vi "Mavlink Initialize.vi"(7 "error in":errorcluster, 9 "Packet Sequence In":u8, 10 "VISA in":refnum<visa-resource-name>) -> (0 "Error Out":errorcluster, 2 "Packet Sequence Out":u8, 3 "VISA resource name Out":refnum<visa-resource-name>)   [LabVIEW 2023]
panel:
  out "Send Data":string
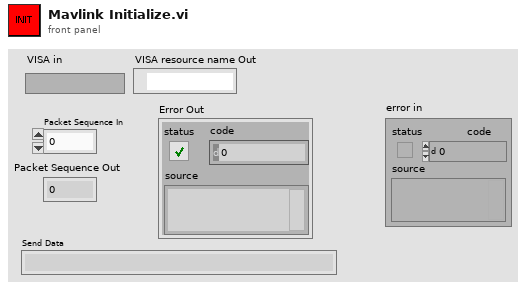
[diagram p1: front panel]
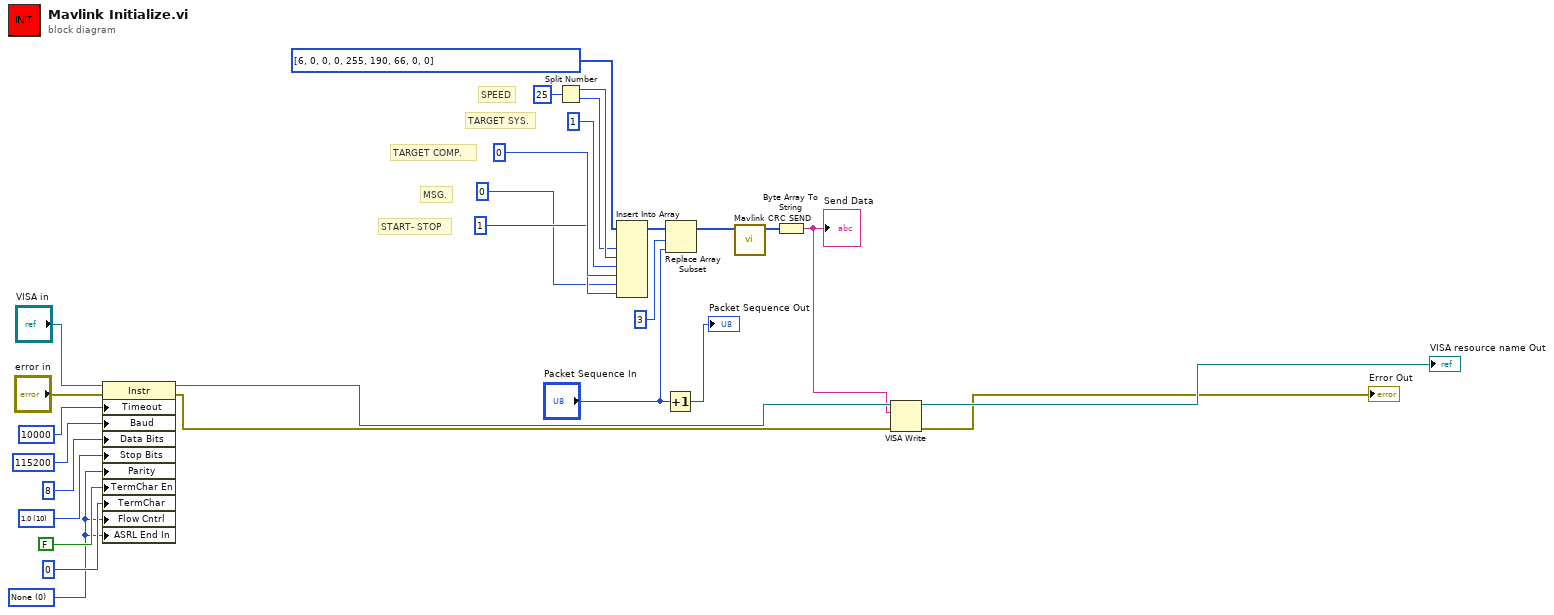
[diagram p0: block diagram]
diagram:
  w20 = u16 0 items=["None", "Last Bit", "TermChar"] ("Serial Settings:End Mode for Reads")
  w23 = u16 10 items=["1.0"=10, "1.5"=15, "2.0"=20] ("Serial Settings:Stop Bits")
  # "START- STOP"
  # "TARGET COMP."
  # "TARGET SYS."
  # "SPEED"
  # "MSG."
  n1 = property class="Instr"(reference="VISA in", error in="error in", "Timeout"=u32 10000 ("General Settings:Timeout Value"), "Baud"=u32 115200 ("Serial Settings:Baud Rate"), "Data Bits"=u16 8 ("Serial Settings:Data Bits"), "Stop Bits"=w23, "Parity"=w20, "TermChar En"=FALSE ("Message Based Settings:Termination Character Enable"), "TermChar"=u8 0 ("Message Based Settings:Termination Character"), "Flow Cntrl"=w20, "ASRL End In"=w20) -> (reference out=w17:refnum<visa-resource-name>, error out=w16:errorcluster)
  n2 = Split Number(x=u16 25) -> (hi(x)=w14:u8, lo(x)=w13:u8)
  n3 = Insert Into Array(array=u8[] [6, 0, 0, 0, 255, 190, 66, 0, 0] ("milliseconds to wait"), new element #1=w13, new element #2=w14, new element #3=u8 1, new element #4=u8 0, new element #5=u8 0 ("new element/subarray"), new element #6=u8 1) -> (w7:u8[])  [unwired: 1 in]
  n4 = Increment(x="Packet Sequence In") -> (x+1=→"Packet Sequence Out":u8)
  n5 = Replace Array Subset(array=w7, new element="Packet Sequence In", index=3) -> (w6:u8[])
  n6 = call "Mavlink CRC SEND.vi"("Byte In"=w6) -> ("Output Byte"=w5:u8[])  [unwired: 10 in]
  n7 = Byte Array To String(unsigned byte array=w5) -> (string=w1:string)
  "Send Data" <- w1
  n8 = VISA Write(VISA resource name=w17, write buffer=w1, error in (no error)=w16) -> (VISA resource name out=→"VISA resource name Out":refnum<visa-resource-name>, error out=→"Error Out":errorcluster)  [unwired: 1 out]
